vi "LimitReached.vi"(8 "error in (no error)":errorcluster, 11 "InterferometrUI in":refnum<class "InterferometerUI.lvclass">) -> (0 "error out":errorcluster, 3 "InterferometrUI out":refnum<class "InterferometerUI.lvclass">)   [LabVIEW 2023, in "InterferometrUI.lvlib" / "InterferometerUI.lvclass"]
uses:
  InterferometerUI.lvclass
  InterferometerUI.lvclass/InterferometerUI.ctl
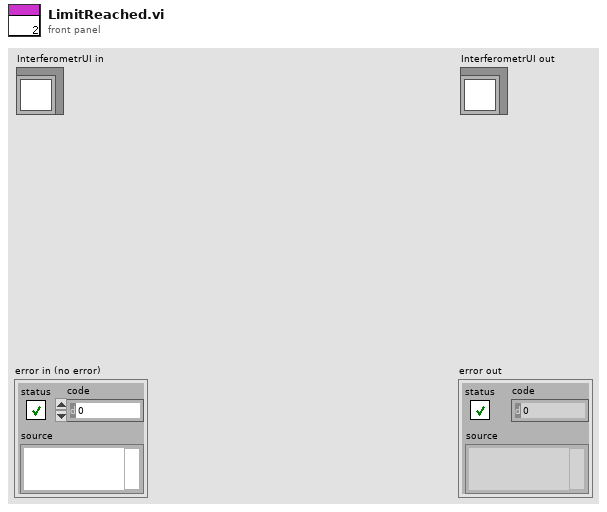
[diagram p1: front panel]
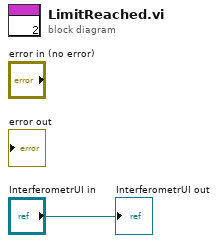
[diagram p0: block diagram]
diagram:
  "InterferometrUI out" <- "InterferometrUI in"
